vi "MT Generate QAM Symbol Map.vi"(0 "symbol values":i32[][](array[numeric]), 11 "error in (no error)":errorcluster) -> (4 "symbol map":cdb[](array[numeric]) format="%.3f", 6 "bits per symbol":i32, 15 "error out":errorcluster)   [LabVIEW 2020, in "niDMT.lvlib"]
uses:
  <vilib>/addons/Modulation/niDMT.lvlib
  <vilib>/addons/Modulation/niAMT.lvlib
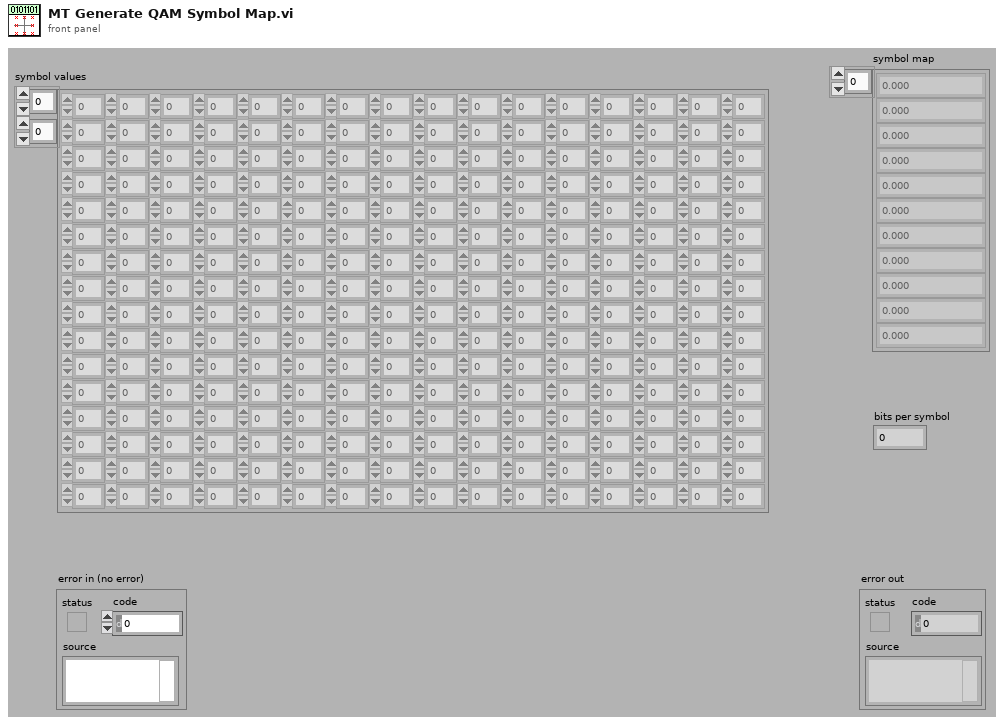
[diagram p1: front panel]
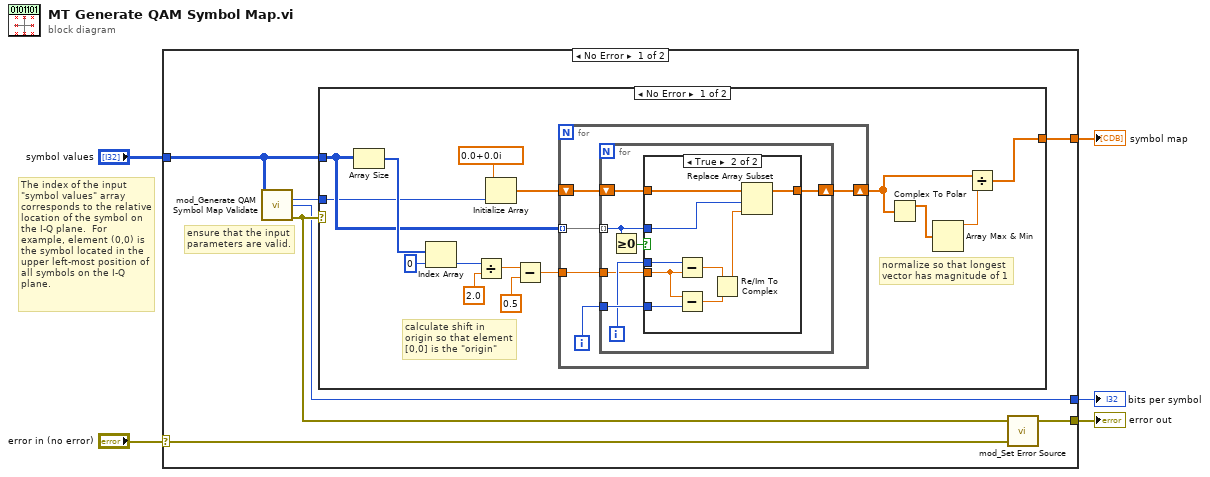
[diagram p0: block diagram]
diagram:
  # "The index of the input \"symbol values\" array corresponds to the relative location of the symbol on the I-Q plane.  For example, element (0,0) is the symbol located in the upper left-most position of all symbols on the I-Q plane."
  n1 = case shown="No Error" "error in (no error)" {
    selector: "error in (no error)" -> [w12 w50]
    tunnel: "symbol values" -> [w10 _]
    tunnel: [w11 w50] -> w4
    tunnel: [w9 _] -> w2
    tunnel: [w6 _] -> w1
    frame No Error {
      # "ensure that the input parameters are valid."
      n2 = call <vilib>:"mod_Generate QAM Symbol Map Validate.vi"("Symbol Values"=w10) -> ("# of values"=w7:i32, "bits per symbol"=w6:i32, "error out"=w8:errorcluster)  [unwired: 12 out]
      n3 = case shown="No Error" w8 {
        tunnel: w10 -> [w16 _]
        tunnel: [w14 _] -> w9
        tunnel: w7 -> [w15 _]
        frame No Error {
          # "calculate shift in origin so that element [0,0] is the \"origin\""
          # "normalize so that longest vector has magnitude of 1"
          n4 = Array Size(array=w16) -> (size(s)=w27:i32[])
          n5 = Index Array(array=w27, index=0) -> (element=w22:i32)
          n6 = Divide(x=w22, y=2.0) -> (x/y=w24:dbl)
          n7 = Initialize Array(cdb 0.0+0.0i, w15) -> (w19:cdb[])
          n8 = Subtract(x=w24, y=0.5) -> (x-y=w21:dbl)
          n9 = for {
            tunnel: w16 -> [w32] mode=indexing
            shift-right: [w28] -> w13
            shift-left: w19 -> [w31]
            tunnel: w21 -> [w29]
            i -> [w30]
            n10 = for {
              tunnel: w32 -> [w34] mode=indexing
              shift-right: [w36] -> w28
              shift-left: w31 -> [w35]
              tunnel: w30 -> [w39]
              tunnel: w29 -> [w37]
              i -> [w38]
              n11 = Greater Or Equal To 0?(x=w34) -> (x >= 0?=w33:bool)
              n12 = case shown="True" w33 {
                tunnel: w39 -> [_ w49]
                tunnel: w38 -> [_ w48]
                tunnel: w37 -> [_ w47]
                tunnel: [w40 w44] -> w36
                tunnel: w35 -> [w40 w43]
                tunnel: w34 -> [_ w42]
                frame False {
                }
                frame True {
                  n13 = Subtract(x=w48, y=w47) -> (x-y=w46:dbl)
                  n14 = Subtract(x=w47, y=w49) -> (x-y=w45:dbl)
                  n15 = Re/Im To Complex(1:w45, 2:w46) -> (0:w41:cdb)
                  n16 = Replace Array Subset(array=w43, new element=w41, index=w42) -> (w44:cdb[])
                }
              }
            }
          }
          n17 = Complex To Polar(r * e^(i*theta)=w13) -> (r=w18:dbl[])  [unwired: 1 out]
          n18 = Array Max & Min(array=w18) -> (max value=w17:dbl)  [unwired: 3 out]
          n19 = Divide(x=w13, y=w17) -> (x/y=w14:cdb[])
        }
        frame Error {
        }
      }
      n20 = call <vilib>:"mod_Set Error Source.vi"("initial error in (no error)"=w12, "final error in (no error)"=w8) -> ("error out"=w11:errorcluster)  [unwired: 3 out]
    }
    frame Error {
    }
  }
  "error out" <- w4
  "symbol map" <- w2
  "bits per symbol" <- w1
